vi "List Test Node MAC.vi"(8 "error in (no error)":errorcluster, 10 "Edit Test Node List":string[](array[string]), 11 "Edit Test Node View in":refnum<class "Edit Test Node View.lvclass">) -> (0 "error out":errorcluster, 3 "Edit Test Node View out":refnum<class "Edit Test Node View.lvclass">)   [LabVIEW 2013, in "Edit Test Node View.lvlib" / "Edit Test Node View.lvclass"]
uses:
  Edit Test Node View.lvclass
  Edit Test Node View.lvclass/Edit Test Node View.ctl
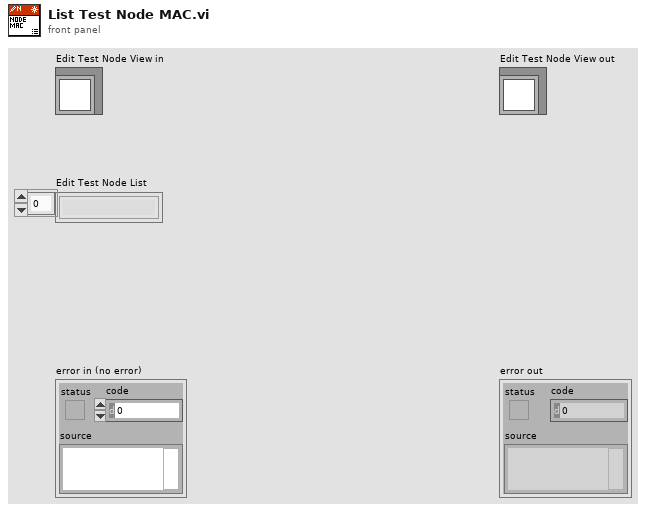
[diagram p1: front panel]
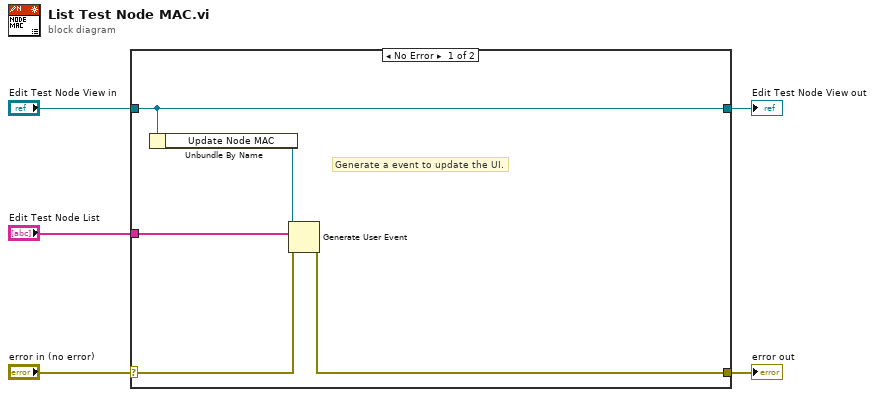
[diagram p0: block diagram]
diagram:
  n1 = case shown="No Error" "error in (no error)" {
    selector: "error in (no error)" -> [w7 w12]
    tunnel: [w6 w12] -> w4
    tunnel: [w10 w11] -> w2
    tunnel: "Edit Test Node View in" -> [w10 w11]
    tunnel: "Edit Test Node List" -> [w8 _]
    frame No Error {
      # "Generate a event to update the UI."
      n2 = Unbundle By Name(w10) -> ("Update Node MAC"=w9:refnum<user-event>)
      n3 = Generate User Event(user event=w9, event data cluster=w8, error in=w7) -> (error out=w6:errorcluster)  [unwired: 1 in, 1 out]
    }
    frame Error {
    }
  }
  "error out" <- w4
  "Edit Test Node View out" <- w2
